vi "Apply Opacity.vi"(7 "% (100)":u8=100, 9 "Bottom":picture, 11 "Top":picture) -> (3 "new picture":picture)   [LabVIEW 2020, in "lv_icon.lvlib"]
doc: "Merge two glyphs and apply a certain opacity to the Top glyph.s"
uses:
  <vilib>/LabVIEW Icon API/lv_icon/lv_icon.lvlib
  <vilib>/picture/picture.llb/Draw True-Color Pixmap.vi
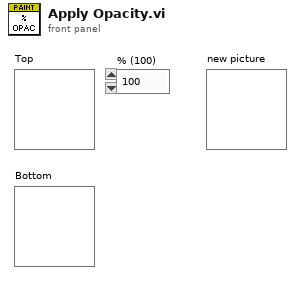
[diagram p1: front panel]
types:
  T1 = cluster{"left":i16, "top":i16, "right":i16, "bottom":i16}
  T2 = typedef "imagedata.ctl" = cluster{"image type":i32, "image depth":i32, "image":u8[], "mask":u8[], "colors":u32[], "Rectangle":cluster{"left":i16, "top":i16, "right":i16, "bottom":i16}}
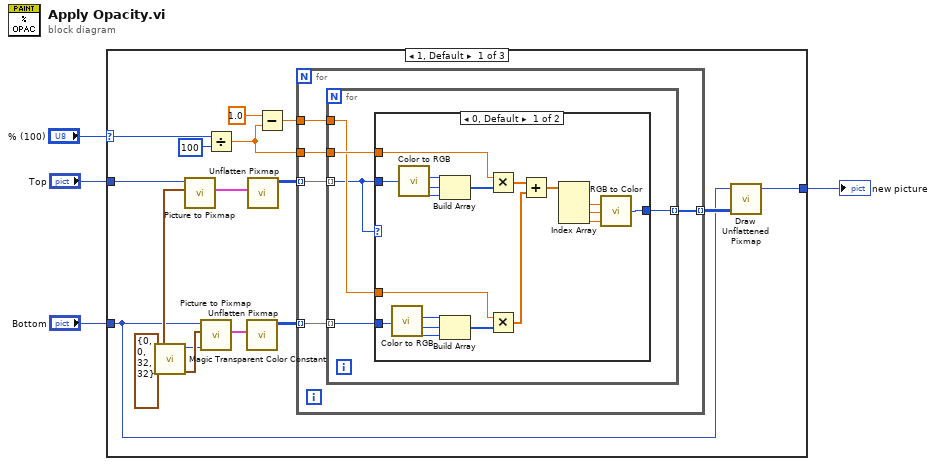
[diagram p0: block diagram]
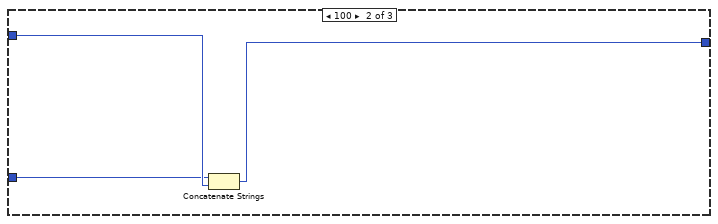
[diagram p3: hidden frame]
diagram:
  n1 = case shown="1, Default" "% (100)" {
    selector: "% (100)" -> [w8 _ _]
    tunnel: [w6 w50 w53] -> w1
    tunnel: "Bottom" -> [w7 w51 w53]
    tunnel: "Top" -> [w13 w52 _]
    frame 1, Default {
      w11 = T1 {"left"=0, "top"=0, "right"=32, "bottom"=32} ("rect")
      n2 = call <vilib>:"Magic Transparent Color Constant.vi"() -> ("Magic transparent color constant"=w5:u32)  [unwired: 11 out]
      n3 = call <vilib>:"Picture to Pixmap.vi"("rect"=w11, "picture"=w13) -> ("image data"=w12:T2)  [unwired: 2 in, 7 out]
      n4 = call <vilib>:"Picture to Pixmap.vi"("Background Color"=w5, "rect"=w11, "picture"=w7) -> ("image data"=w14:T2)  [unwired: 1 in, 7 out]
      n5 = Divide(x=w8, y=u8 100) -> (x/y=w9:dbl)
      n6 = call <vilib>:"Unflatten Pixmap.vi"("image data"=w14) -> ("24-bit pixmap"=w16:u32[][])  [unwired: 10 out]
      n7 = call <vilib>:"Unflatten Pixmap.vi"("image data"=w12) -> ("24-bit pixmap"=w15:u32[][])  [unwired: 10 out]
      n8 = Subtract(x=1.0, y=w9) -> (x-y=w17:dbl)
      n9 = for {
        tunnel: w15 -> [w24] mode=indexing
        tunnel: w9 -> [w23]
        tunnel: [w22] -> w19 mode=indexing
        tunnel: w17 -> [w21]
        tunnel: w16 -> [w20] mode=indexing
        n10 = for {
          tunnel: w24 -> [w25] mode=indexing
          tunnel: w23 -> [w29]
          tunnel: [w28] -> w22 mode=indexing
          tunnel: w21 -> [w26]
          tunnel: w20 -> [w27] mode=indexing
          n11 = case shown="0, Default" w25 {
            tunnel: w29 -> [w44 _]
            tunnel: [w40 w49] -> w28
            tunnel: w27 -> [w35 w49]
            tunnel: w26 -> [w34 _]
            tunnel: w25 -> [w30 _]
            frame 0, Default {
              n12 = call <vilib>:"Color to RGB.vi"("Color"=w35) -> ("R"=w38:u8, "G"=w37:u8, "B"=w36:u8)  [unwired: 1 out]
              n13 = call <vilib>:"Color to RGB.vi"("Color"=w30) -> ("R"=w46:u8, "G"=w47:u8, "B"=w48:u8)  [unwired: 1 out]
              n14 = Build Array(w46, w47, w48) -> (w45:u8[])
              n15 = Build Array(w38, w37, w36) -> (w39:u8[])
              n16 = Multiply(x=w44, y=w45) -> (x*y=w33:dbl[])
              n17 = Multiply(x=w34, y=w39) -> (x*y=w32:dbl[])
              n18 = Add(x=w33, y=w32) -> (x+y=w31:dbl[])
              n19 = Index Array(array=w31) -> (element #1=w42:dbl, element #2=w43:dbl, element #3=w41:dbl)  [unwired: 3 in]
              n20 = call <vilib>:"RGB to Color.vi"("B"=w41, "G"=w43, "R"=w42) -> ("Color"=w40:u32)
            }
            frame 16777215 {
              # "True White color"
            }
          }
        }
      }
      n21 = call-poly <vilib>:"Draw Unflattened Pixmap.vi"("picture"=w7, "data (RGB format)"=w19) -> ("new picture"=w6:picture)  [unwired: 2 in, 5 out]
    }
    frame 100 {
      n22 = Concatenate Strings(w51, w52) -> (w50:picture)
    }
    frame 0 {
    }
  }
  "new picture" <- w1
